vi "GetFontKeys.vi"(5 "name":string, 9 "Font":T2) -> (3 "font items":T1[](array[typedef]))   [LabVIEW 2014, in "Raspberry Pi Compatible Compiler for LabVIEW.lvlib" / "PythonConverter_GUI.lvclass"]
uses:
  PythonConverter_GUI.lvclass
  <vilib>/Utility/miscctls.llb/LVFontTypeDef.ctl
  PythonConfiguration/TypeDefs/ItemTD.ctl
  PythonConfiguration/PythonConfiguration.lvclass
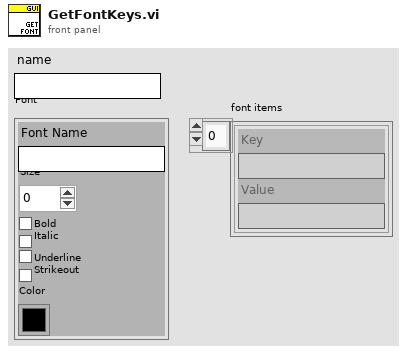
[diagram p1: front panel]
types:
  T1 = typedef "Raspberry Pi Compatible Compiler for LabVIEW.lvlib/PythonConfiguration.lvclass/ItemTD.ctl" = cluster{"Key":string, "Value":string}
  T2 = typedef "LVFontTypeDef.ctl" = cluster{"Font Name":string, "Size":u16, "Bold":bool, "Italic":bool, "Underline":bool, "Strikeout":bool, "Color":u32}
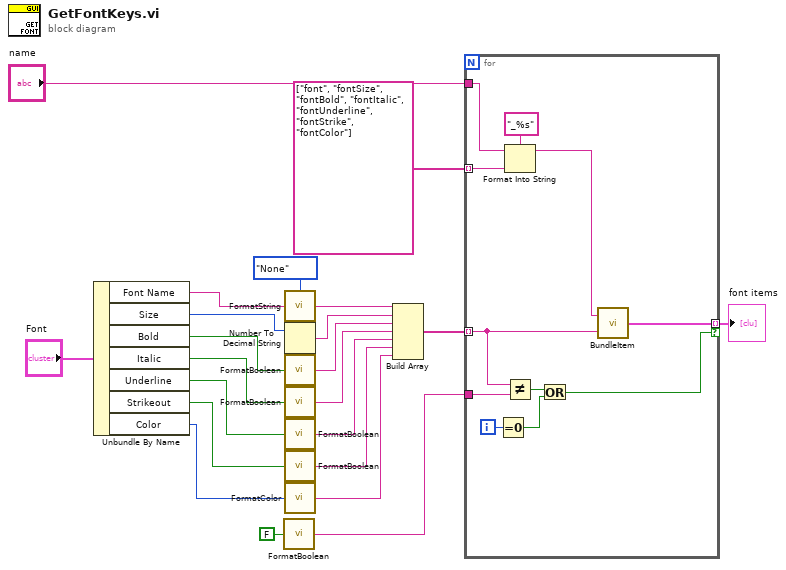
[diagram p0: block diagram]
diagram:
  n1 = Unbundle By Name("Font") -> ("Font Name"=w21:string, "Size"=w19:u16, "Bold"=w18:bool, "Italic"=w17:bool, "Underline"=w16:bool, "Strikeout"=w15:bool, "Color"=w14:u32)
  n2 = call "FormatBoolean.vi"("boolean"=FALSE) -> ("value"=w1:string)
  n3 = call "FormatString.vi"("String"=w21, "string encoding"=enum16{"None", "Base64"}."None") -> ("value"=w13:string)
  n4 = Number To Decimal String(number=w19) -> (decimal integer string=w12:string)  [unwired: 1 in]
  n5 = call "FormatBoolean.vi"("boolean"=w18) -> ("value"=w11:string)
  n6 = call "FormatBoolean.vi"("boolean"=w17) -> ("value"=w10:string)
  n7 = call "FormatBoolean.vi"("boolean"=w16) -> ("value"=w9:string)
  n8 = call "FormatBoolean.vi"("boolean"=w15) -> ("value"=w8:string)
  n9 = call "FormatColor.vi"("color"=w14) -> ("value"=w7:string)
  n10 = Build Array(w13, w12, w11, w10, w9, w8, w7) -> (w4:string[])
  n11 = for {
    tunnel: string[] ["font", "fontSize", "fontBold", "fontItalic", "fontUnderline", "fontStrike", "fontColor"] -> [w33] mode=indexing
    tunnel: "name" -> [w32]
    tunnel: w4 -> [w27] mode=indexing
    tunnel: [w29] -> w3 mode=indexing if=w23
    tunnel: w1 -> [w26]
    i -> [w28]
    n12 = Equal To 0?(x=w28) -> (x = 0?=w24:bool)
    n13 = Format Into String(format string="_%s", initial string=w32, w33) -> (resulting string=w30:string)  [unwired: 1 in, 1 out]
    n14 = Not Equal?(x=w27, y=w26) -> (x != y?=w25:bool)
    n15 = Or(x=w25, y=w24) -> (x .or. y?=w23:bool)
    n16 = call "BundleItem.vi"("Value"=w27, "Key"=w30) -> ("Item"=w29:T1)
  }
  "font items" <- w3
